vi "LV SCISDK Get Components List.vi"(8 "error in (no error)":errorcluster, 9 "handle":u64, 10 "Type":string, 11 "Name":string) -> (0 "error out":errorcluster, 1 "function return":i32, 2 "ret out 2":T1(array[cluster])=[{"path"=" ", "name"="", "type"=""}])   [LabVIEW 2021, in "SciSDK_Labview.lvlib"]
doc: "SCISDKLABVIEW_DLL_API int LV_SCISDK_GetParameterString(char* Path, char* value, void* handle);"
uses:
  SciSDK_Labview.lvlib
  SciSDK_VC++/x64/Debug/SciSDK_Labview.dll
panel:
  in  "ret in":T1(array[cluster])=[{"path"=" ", "name"="", "type"=""}]
  out "handle out":u64
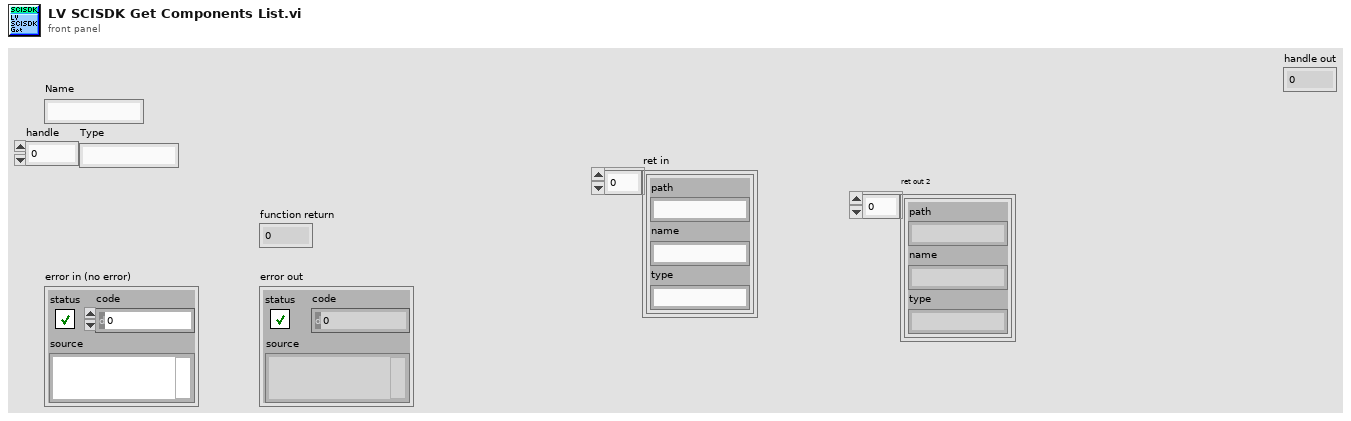
[diagram p1: front panel]
types:
  T1 = cluster{"path":string, "name":string, "type":string}[]
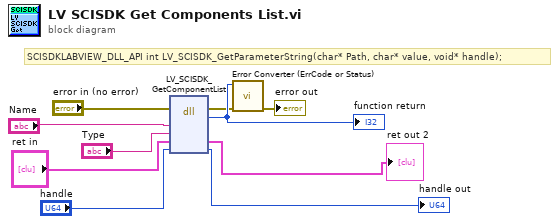
[diagram p0: block diagram]
diagram:
  # "SCISDKLABVIEW_DLL_API int LV_SCISDK_GetParameterString(char* Path, char* value, void* handle);"
  n1 = dll-call lib="C:/git/scisdk/SciSDK_VC++/x64/Debug/SciSDK_Labview.dll" fn="LV_SCISDK_GetComponentList"(error in="error in (no error)", "Path"="Name", "type"="Type", "ret"="ret in", "handle"="handle") -> (error out=w7:errorcluster, "return type"=w10:i32, "ret"=→"ret out 2":T1, "handle"=→"handle out":u64)  [unwired: 4 in, 1 out]
  "function return" <- w10
  n2 = call <userlib>:"Error Converter (ErrCode or Status).vi"("error in (no error)"=w7, "error code"=w10) -> ("error out"=→"error out":errorcluster)  [unwired: 9 in]
